vi "Group Check - LogType.vi"(8 "Matched Previous?":bool, 10 "Cross CSM Data (in)":T1={"Name(\"\" to use uuid)"="", "Current State"="", "Arguments"="", "Source Message"={"‘State"="", "’Arguments"="", "’Error"={"status"=FALSE, "code"=0, "source"=""}}, "Source Module"="", "Complete(T)/Start(F)"=FALSE, "LogType"=enum."State Change"}, 11 "GlobalLogFilter.lvclass":refnum<class "LogFilter.lvclass">) -> (0 "Matched? (dup)":bool, 2 "Cross CSM Data":T1={"Name(\"\" to use uuid)"="", "Current State"="", "Arguments"="", "Source Message"={"‘State"="", "’Arguments"="", "’Error"={"status"=FALSE, "code"=0, "source"=""}}, "Source Module"="", "Complete(T)/Start(F)"=FALSE, "LogType"=enum."State Change"}, 3 "GlobalLogFilter.lvclass (dup)":refnum<class "LogFilter.lvclass">)   [LabVIEW 2020, in "Communicable State Machine.lvlib" / "LogFilter.lvclass"]
uses:
  LogFilter.lvclass
  _CSM_GlobalLog_MSG.ctl
  _CSM_Response Source Message.ctl
  _CSM_GlobalLog_MSG_TYPE.ctl
  LogFilter.lvclass/LogFilter.ctl
  Communicable State Machine.lvlib
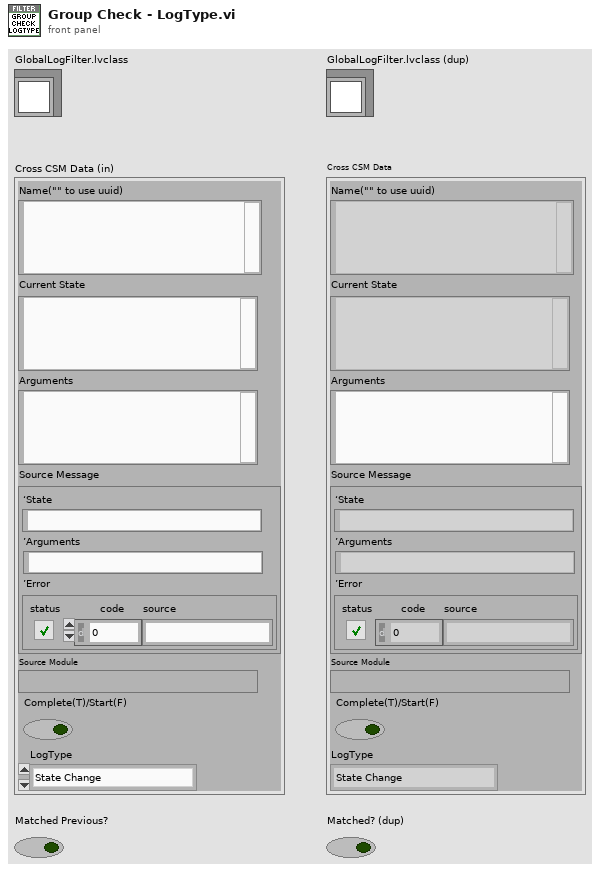
[diagram p1: front panel]
types:
  T1 = typedef "Communicable State Machine.lvlib/_CSM_GlobalLog_MSG.ctl" = cluster{"Name(\"\" to use uuid)":string, "Current State":string, "Arguments":string, "Source Message":T2, "Source Module":string, "Complete(T)/Start(F)":bool, "LogType":T3}
  T2 = typedef "Communicable State Machine.lvlib/_CSM_Response Source Message.ctl" = cluster{"‘State":string, "’Arguments":string, "’Error":errorcluster}
  T3 = typedef "Communicable State Machine.lvlib/_CSM_GlobalLog_MSG_TYPE.ctl" = enum16{"User Log", "State Change", "Status", "Interrupt", "Register", "Unregister", "Error Log", "Module Created", "Module Destroyed"}
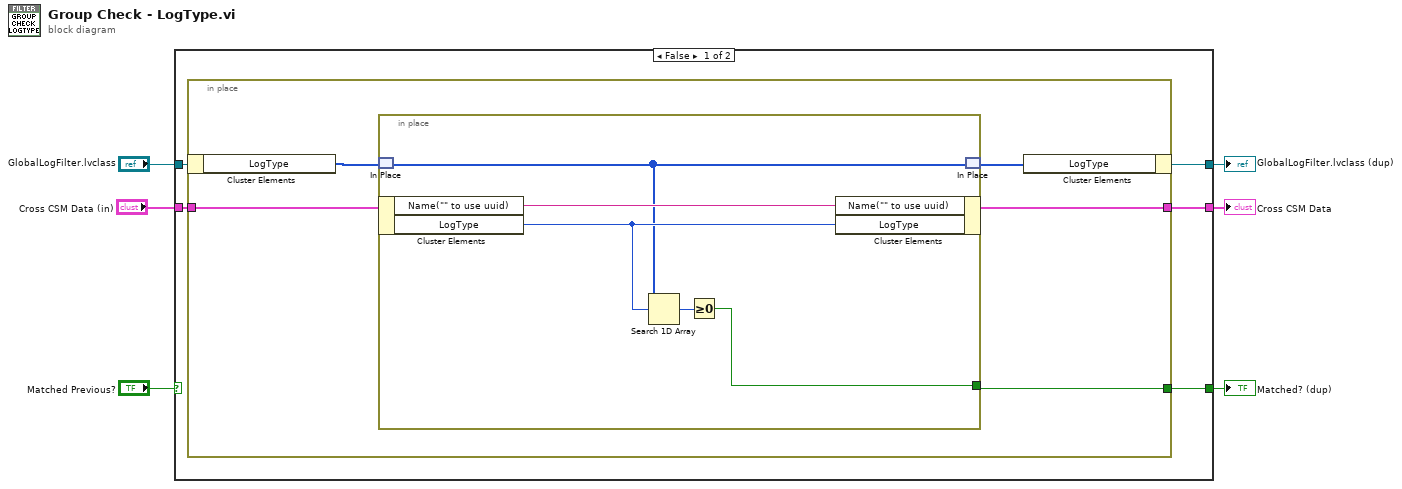
[diagram p0: block diagram]
diagram:
  n1 = case shown="False" "Matched Previous?" {
    selector: "Matched Previous?" -> [_ w23]
    tunnel: [w10 w24] -> w5
    tunnel: "Cross CSM Data (in)" -> [w11 w24]
    tunnel: [w9 w23] -> w3
    tunnel: [w7 w22] -> w2
    tunnel: "GlobalLogFilter.lvclass" -> [w8 w22]
    frame False {
      n2 = in-place {
        in-place-border: w11 -> [w16]
        in-place-border: [w15] -> w10
        in-place-border: [w14] -> w9
        n3 = in-place-cluster #1(w8) -> ("LogType"=w13:T3[])
        n4 = in-place {
          in-place-border: [w18] -> w14
          n5 = in-place-match #2(w13) -> (w17:T3[])
          n6 = in-place-cluster #3(w16) -> ("Name(\"\" to use uuid)"=w21:string, "LogType"=w20:T3)
          n7 = Search 1D Array(1D array=w17, element=w20) -> (index of element=w19:i32)  [unwired: 1 in]
          n8 = Greater Or Equal To 0?(x=w19) -> (x >= 0?=w18:bool)
          n9 = in-place-cluster #3("Name(\"\" to use uuid)"=w21, "LogType"=w20) -> (w15:T1)
          n10 = in-place-match #2(w17) -> (w12:T3[])
        }
        n11 = in-place-cluster #1("LogType"=w12) -> (w7:refnum<class "LogFilter.lvclass">)
      }
    }
    frame True {
    }
  }
  "Cross CSM Data" <- w5
  "Matched? (dup)" <- w3
  "GlobalLogFilter.lvclass (dup)" <- w2
